vi "head.vi"(7 "transmit queue":refnum<queue>, 10 "application request in":T1, 11 "test responder in":refnum<class "test responder.lvclass">) -> (0 "error out":errorcluster, 3 "test responder out":refnum<class "test responder.lvclass">)   [LabVIEW 2013, in "test responder.lvclass"]
uses:
  test responder.lvclass
  HTTP server/http response.ctl
  HTTP server/http response packet type.ctl
  HTTP headers/http header data.ctl
  HTTP server/http request.ctl
  HTTP server/http method.ctl
  URI/url structure.ctl
  HTTP responder/http responder.lvclass
  HTTP server/Basic HTTP server.lvclass
  HTTP headers/http headers.lvlib
  URI/uniform resource locator.lvlib
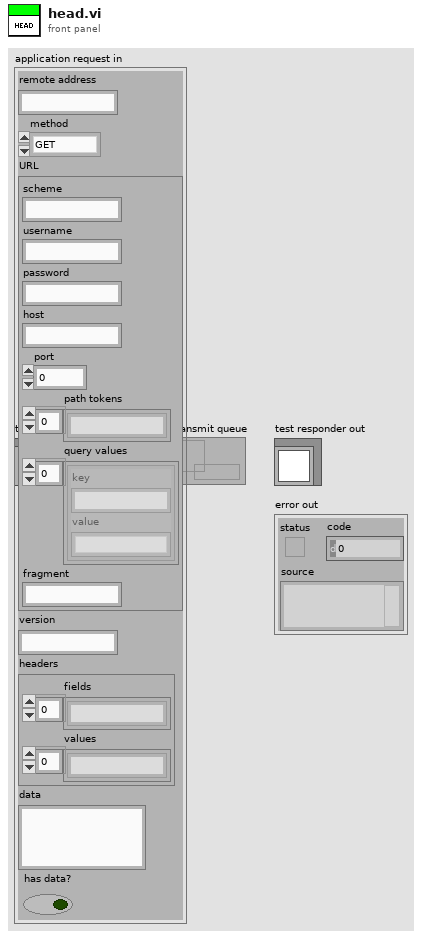
[diagram p1: front panel]
types:
  T1 = typedef "Basic HTTP server.lvclass/http request.ctl" = cluster{"remote address":string, "method":T2, "URL":T3, "version":string, "headers":T4, "data":string, "has data?":bool}
  T2 = typedef "Basic HTTP server.lvclass/http method.ctl" = enum16{"GET", "POST", "PUT", "DELETE", "HEAD", "OPTIONS", "upgrade"}
  T3 = typedef "uniform resource locator.lvlib/url structure.ctl" = cluster{"scheme":string, "username":string, "password":string, "host":string, "port":u16, "path tokens":string[], "query values":cluster{"key":string, "value":string}[], "fragment":string}
  T4 = typedef "http headers.lvlib/http header data.ctl" = cluster{"fields":string[], "values":string[]}
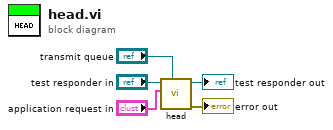
[diagram p0: block diagram]
diagram:
  n1 = call-parent "head.vi"("transmit queue"="transmit queue", "application request in"="application request in", "http responder in"="test responder in") -> ("error out"=→"error out":errorcluster, "http responder out"=→"test responder out":refnum<class "test responder.lvclass">)  [unwired: 7 in]
